vi "Write QueueSerial.vi"(8 "error in (no error)":errorcluster, 10 "QueueSerial":refnum<queue>, 11 "StateAuto in":refnum<class "StateAuto.lvclass">) -> (0 "error out":errorcluster, 3 "StateAuto out":refnum<class "StateAuto.lvclass">)   [LabVIEW 2017, in "LibraryGcode.lvlib" / "StateAuto.lvclass"]
uses:
  StateAuto.lvclass
  StateAuto.lvclass/StateAuto.ctl
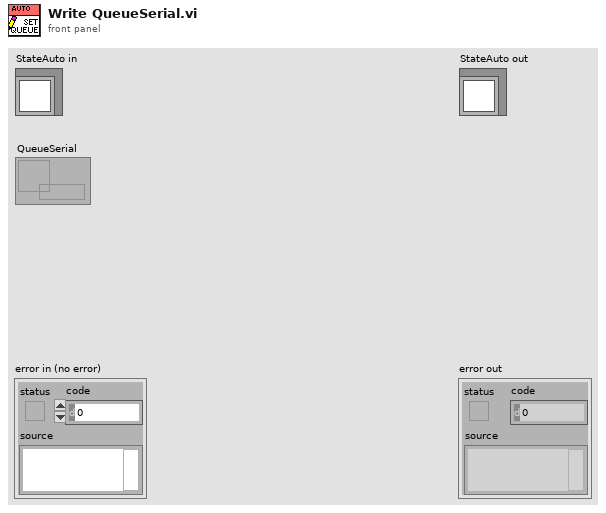
[diagram p1: front panel]
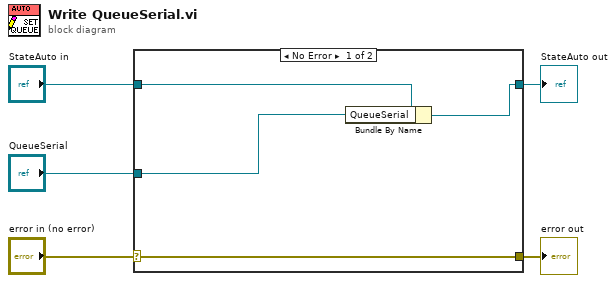
[diagram p0: block diagram]
diagram:
  n1 = case shown="No Error" "error in (no error)" {
    selector: "error in (no error)" -> [w9 w10]
    tunnel: [w9 w10] -> w4
    tunnel: [w7 w11] -> w2
    tunnel: "StateAuto in" -> [w8 w11]
    tunnel: "QueueSerial" -> [w6 _]
    frame No Error {
      n2 = Bundle By Name(cluster=w8, "QueueSerial"=w6) -> (w7:refnum<class "StateAuto.lvclass">)
    }
    frame Error {
    }
  }
  "error out" <- w4
  "StateAuto out" <- w2
